vi "Find Baseplate Center.vi"() -> ()   [LabVIEW 2019]
uses:
  Classes/Workspace/Workspace.ctl
  Classes/Workspace/Carrier Tray/Assembly Tray.lvclass
  Classes/Controller/Controller.lvclass
  Classes/Workspace/Fixture.lvclass
panel:
  out "error out":errorcluster
  out "Workspace":T1
  in  "error in (no error)":errorcluster
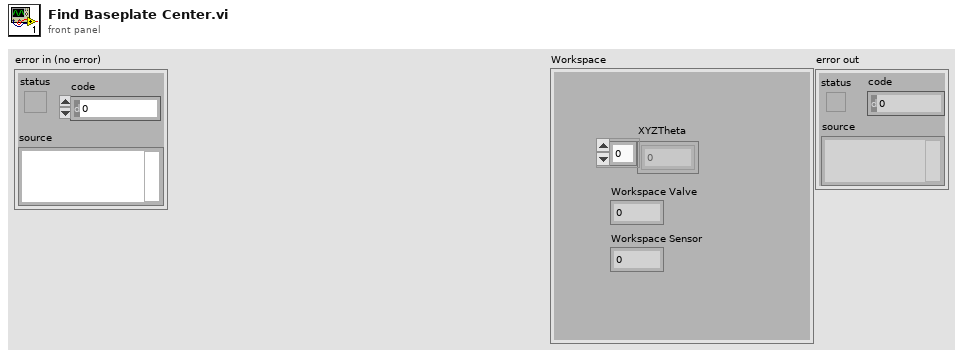
[diagram p1: front panel]
types:
  T1 = typedef "Fixture.lvclass/Workspace.ctl" = cluster{"XYZTheta":dbl[], "Workspace Valve":i32, "Workspace Sensor":i32}
  T2 = typedef "Controller.lvclass/Controllers.ctl" = cluster{"I-O.lvclass":refnum<class "I-O.lvclass">, "Dispenser.lvclass":refnum<class "Dispenser.lvclass">, "Gantry":refnum<k24>}
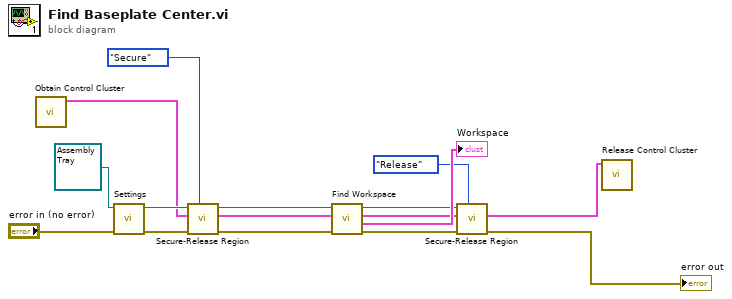
[diagram p0: block diagram]
diagram:
  n1 = call "Obtain Control Cluster.vi"() -> ("Control Out"=w12:T2)  [unwired: 11 in]
  n2 = call-dynamic "Settings.vi"("error in (no error)"="error in (no error)", "Assembly Tray In"=refnum<class "Assembly Tray.lvclass"> refnum ("Assembly Tray.lvclass")) -> ("error out"=w14:errorcluster, "Assembly Tray Out"=w15:refnum<class "Assembly Tray.lvclass">)  [unwired: 8 in]
  n3 = call-dynamic "Secure-Release Region.vi"("Action"=enum16{"Secure", "Release"}."Secure", "error in (no error)"=w14, "Control In"=w12, "Carrier Tray in"=w15) -> ("error out"=w8:errorcluster, "Control Out"=w9:T2, "Carrier Tray out"=w10:refnum<class "Assembly Tray.lvclass">)  [unwired: 5 in]
  n4 = call-dynamic "Find Workspace.vi"("Error In"=w8, "Control In"=w9, "Carrier Tray in"=w10) -> ("Error Out"=w4:errorcluster, "Workspace"=→"Workspace":T1, "Control Out"=w5:T2, "Carrier Tray Out"=w6:refnum<class "Assembly Tray.lvclass">)  [unwired: 5 in]
  n5 = call-dynamic "Secure-Release Region.vi"("Action"=enum16{"Secure", "Release"}."Release", "error in (no error)"=w4, "Control In"=w5, "Carrier Tray in"=w6) -> ("error out"=→"error out":errorcluster, "Control Out"=w3:T2)  [unwired: 5 in, 1 out]
  n6 = call "Release Control Cluster.vi"("output cluster"=w3) -> ()  [unwired: 11 in]
